vi "Write Icon.vi"(8 "error in (no error)":errorcluster, 9 "Icon":T1, 11 "Grove I2C Matrix LED in":refnum<class "Grove I2C Matrix LED Driver.lvclass">) -> (0 "error out":errorcluster, 3 "Grove I2C Matrix LED out":refnum<class "Grove I2C Matrix LED Driver.lvclass">)   [LabVIEW 2020, in "CTI-Peripheral.lvlib" / "Grove I2C Matrix LED Driver.lvclass"]
uses:
  Grove I2C Matrix LED Driver.lvclass
  Grove I2C Matrix LED Driver.lvclass/Grove I2C Matrix LED Driver.ctl
  CTI/I2C Connection/I2C Connection.lvclass
  Base/Data Types/ICONS.ctl
  Base/LEDMatrix.lvclass
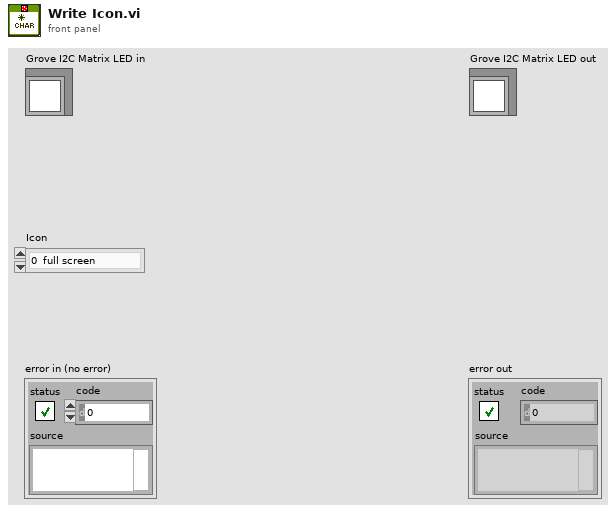
[diagram p1: front panel]
types:
  T1 = typedef "CTI-Peripheral.lvlib/LEDMatrix.lvclass/ICONS.ctl" = enum16{"0  full screen", "1  arrow_up", "2  arrow_down", "3  arrow_right", "4  arrow_left", "5  triangle_up", "6  triangle_down", "7  triangle_right", "8  triangel_left", "9  smile_face_1", "10 smile_face_2", "11 hearts", "12 diamonds", "13 clubs", "14 spades", "15 circle1", "16 circle2", "17 circle3", "18 circle4", "19 man", "20 woman", "21 musical_note_1", "22 musical_note_2", "23 snow", "24 up_down", "25 double_!", "26 left_right", "27 house"}
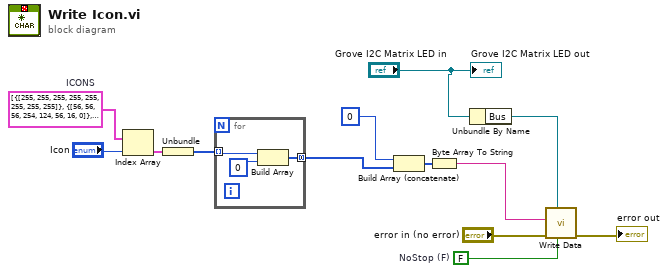
[diagram p0: block diagram]
diagram:
  w4 = cluster{"BytesOut":u8[]}[] [{"BytesOut"=[255, 255, 255, 255, 255, 255, 255, 255]}, {"BytesOut"=[56, 56, 56, 254, 124, 56, 16, 0]}, {"BytesOut"=[16, 56, 124, 254, 56, 56, 56, 0]}, {"BytesOut"=[16, 48, 126, 254, 126, 48, 16, 0]}, {"BytesOut"=[16, 24, 252, 254, 252, 24, 16, 0]}, {"BytesOut"=[254, 254, 124, 124, 56, 56, 16, 0]}, {"BytesOut"=[16, 56, 56, 124, 124, 254, 254, 0]}, {"BytesOut"=[6, 30, 126, 254, 126, 30, 6, 0]}, {"BytesOut"=[192, 240, 252, 254, 252, 240, 192, 0]}, {"BytesOut"=[124, 146, 170, 130, 170, 130, 124, 0]}, {"BytesOut"=[0, 60, 66, 0, 0, 102, 0, 0]}, {"BytesOut"=[16, 56, 124, 254, 254, 238, 68, 0]}, {"BytesOut"=[16, 56, 124, 254, 124, 56, 16, 0]}, {"BytesOut"=[56, 16, 84, 254, 84, 56, 16, 0]}, {"BytesOut"=[56, 16, 124, 254, 124, 56, 16, 0]}, {"BytesOut"=[0, 56, 124, 124, 124, 56, 0, 0]}, {"BytesOut"=[255, 199, 131, 131, 131, 199, 255, 255]}, {"BytesOut"=[0, 56, 68, 68, 68, 56, 0, 0]}, {"BytesOut"=[255, 199, 187, 187, 187, 199, 255, 255]}, {"BytesOut"=[12, 18, 18, 156, 160, 192, 240, 0]}, {"BytesOut"=[56, 68, 68, 56, 16, 124, 16, 0]}, {"BytesOut"=[6, 14, 12, 8, 8, 40, 24, 0]}, {"BytesOut"=[6, 110, 236, 200, 136, 152, 240, 0]}, {"BytesOut"=[16, 84, 56, 238, 56, 84, 16, 0]}, {"BytesOut"=[16, 56, 84, 16, 84, 56, 16, 0]}, {"BytesOut"=[102, 102, 0, 102, 102, 102, 102, 0]}, {"BytesOut"=[0, 40, 68, 254, 68, 40, 0, 0]}, {"BytesOut"=[254, 130, 130, 198, 108, 56, 16, 0]}, {"BytesOut"=[0, 36, 0, 231, 165, 189, 231, 0, 0, 0, 0, 0, 2, 8, 0, 10, 0]}]  # ICONS
  w11 = FALSE  # NoStop (F)
  n1 = Index Array(array=w4, index="Icon") -> (element=w3:cluster{"BytesOut":u8[]})
  n2 = Unbundle(w3) -> ("BytesOut"=w1:u8[])
  n3 = for {
    tunnel: w1 -> [w16] mode=indexing
    tunnel: [w14] -> w6 mode=concatenating
    n4 = Build Array(w16, u8 0 ("Value")) -> (w14:u8[])
  }
  n5 = Build Array (concatenate)(u8 0 ("Value"), w6) -> (w13:u8[])
  n6 = Byte Array To String(unsigned byte array=w13) -> (string=w10:string)
  n7 = Unbundle By Name("Grove I2C Matrix LED in") -> ("Bus"=w9:refnum<class "I2C Connection.lvclass">)
  n8 = call "Write Data.vi"("NoStop (F)"=w11, "I2C Connection"=w9, "error in (no error)"="error in (no error)", "Data"=w10) -> ("error out"=→"error out":errorcluster)  [unwired: 7 in]
  "Grove I2C Matrix LED out" <- "Grove I2C Matrix LED in"
